vi "Read Sensor Type.vi"(8 "error in (no error)":errorcluster, 10 "node address (same)":u8, 11 "ProPar in":refnum<class "PL Bronkhorst ProPar.lvclass">) -> (0 "error out":errorcluster, 2 "sensor type":u8(ring) items=["pressure (controller)"=0, "liquid volume (controller)"=1, "liquid/gas mass (controller)"=2, "gas volume (controller)"=3, "other sensor type (controller)"=4, "pressure (sensor)"=128, "liquid volume (sensor)"=129, "liquid/gas mass (sensor)"=130, "gas volume (sensor)"=131, "other sensor type (sensor)"=132], 3 "ProPar out":refnum<class "PL Bronkhorst ProPar.lvclass">)   [LabVIEW 2015, in "PL Bronkhorst ProPar.lvclass"]
doc: "Reads sensor type of the specified <b>node</b>."
uses:
  PL Bronkhorst ProPar.lvclass
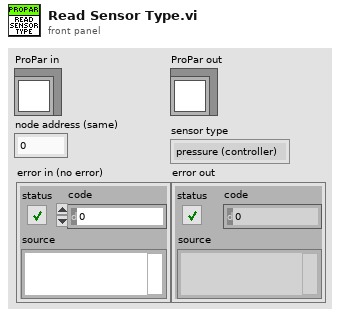
[diagram p1: front panel]
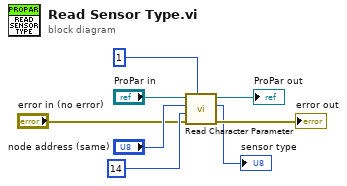
[diagram p0: block diagram]
diagram:
  n1 = call "Read Character Parameter.vi"("process number"=u8 1, "error in (no error)"="error in (no error)", "parameter number"=u8 14 ("process number"), "node address (same)"="node address (same)", "ProPar in"="ProPar in") -> ("error out"=→"error out":errorcluster, "value"=→"sensor type":u8, "ProPar out"=→"ProPar out":refnum<class "PL Bronkhorst ProPar.lvclass">)  [unwired: 4 in]
